vi "emi_ Set VIs Graphs Background .vi"(5 "VI Refnum(This vi)":refnum<vi>, 9 "error in (no error)":errorcluster) -> (6 "VI Refnum":refnum<vi>, 10 "error out":errorcluster)   [LabVIEW 2011]
doc: "Describe...\n\n\nIf no VI ref in, then the VI containing this VI is used.\nIf VI has multiple panes, only the first pane will be used.\n\nOn error in: Does not run."
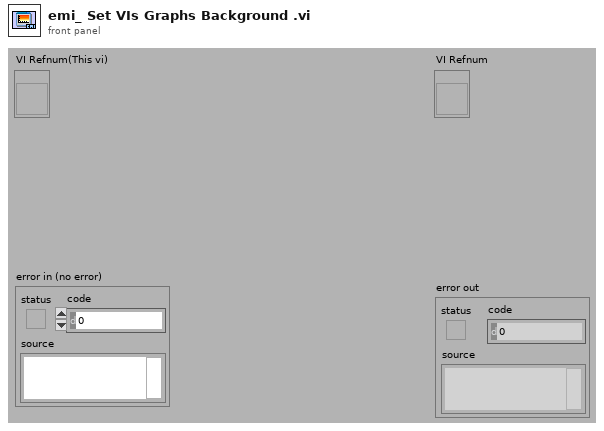
[diagram p1: front panel]
types:
  T1 = typedef "emi_System Colors.ctl" = cluster{"Main Top Panels":T2, "Main Botom Panels":T2, "Graphs":T2, "Dialogs":T2}
  T2 = typedef "_emi_ Color defenition.ctl" = cluster{"Type":T3, "Dark/Primary Color":u32, "Light/Secondary Color":u32, "Extra Color":u32}
  T3 = typedef "emi_List Of Graphix.ctl" = enum16{"FlatColor", "SharpGrad", "ShallowGrad", "GlasGradBord", "GlasGrad", "GlasGradBord 2"}
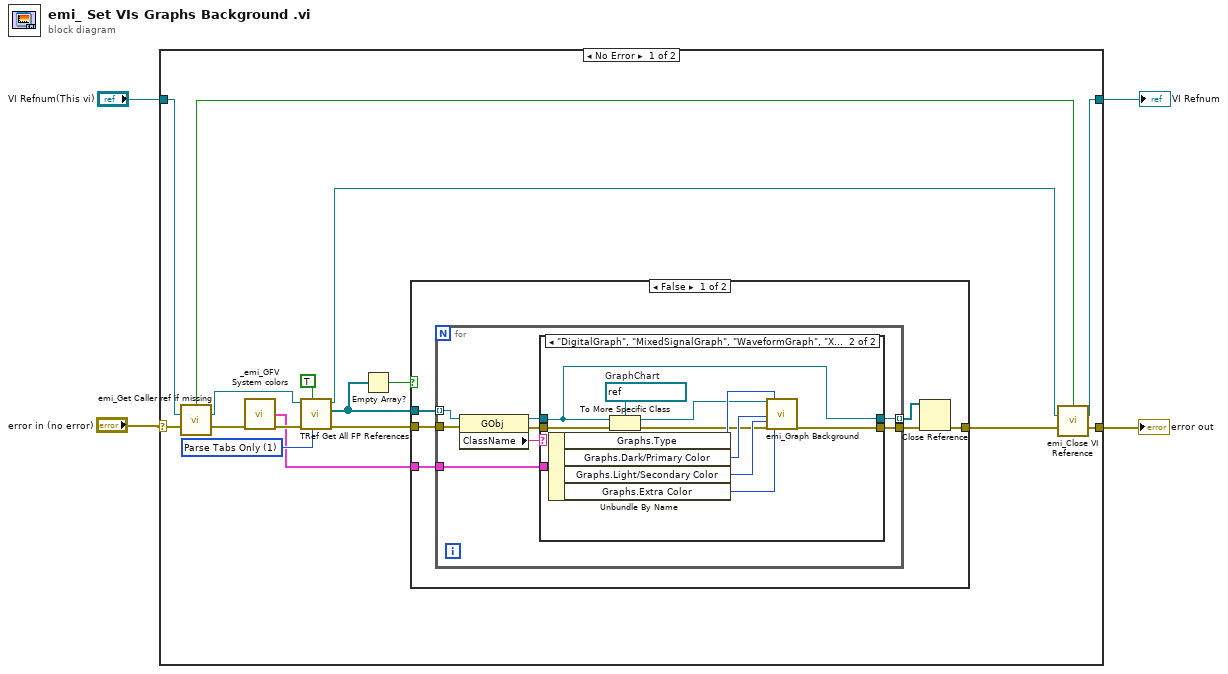
[diagram p0: block diagram]
diagram:
  n1 = case shown="No Error" "error in (no error)" {
    selector: "error in (no error)" -> [w19 w50]
    tunnel: [w17 w50] -> w4
    tunnel: "VI Refnum(This vi)" -> [w18 w49]
    tunnel: [w16 w49] -> w2
    frame No Error {
      w15 = u16 1 items=["Parse All", "Parse Tabs Only"] ("Parsing Rule")
      n2 = call "emi_Get Caller ref if missing.vi"("VI Refnum(Calling VI)"=w18, "error in (no error)"=w19) -> ("Ref Generated"=w20:bool, "VI Refnum Out"=w8:refnum<vi>, "error out"=w7:errorcluster)  [unwired: 11 in]
      n3 = call "_emi_GFV System colors.vi"("error in (no error)"=w7) -> ("System background out"=w9:T1, "error out"=w10:errorcluster)  [unwired: 13 in]
      n4 = call <vilib>:"TRef Get All FP References.vi"("Parsing Rule"=w15, "Ignore Decorations?"=TRUE, "error in (no error)"=w10, "VI Refnum"=w8) -> ("error out"=w11:errorcluster, "All FP Objects"=w12:refnum<vi>[], "dup VI Refnum"=w5:refnum<vi>)  [unwired: 3 in, 2 out]
      n5 = Empty Array?(array=w12) -> (empty?=w13:bool)
      n6 = case shown="False" w13 {
        tunnel: w12 -> [w26 _]
        tunnel: w11 -> [w25 w48]
        tunnel: w9 -> [w24 _]
        tunnel: [w21 w48] -> w6
        frame False {
          n7 = for {
            tunnel: w26 -> [w33] mode=indexing
            tunnel: w25 -> [w34]
            tunnel: w24 -> [w29]
            tunnel: [w28] -> w23
            tunnel: [w27] -> w22 mode=indexing
            n8 = property class="GObj"(reference=w33, error in=w34) -> (reference out=w30:refnum<vi>, error out=w31:errorcluster, "ClassName"=w32:string)
            n9 = case shown="\"DigitalGraph\", \"MixedSignalGraph\", \"WaveformGraph\", \"XYGraph\"" w32 {
              tunnel: w31 -> [w36 w47]
              tunnel: w30 -> [w35 w37]
              tunnel: w29 -> [_ w46]
              tunnel: [w36 w41] -> w28
              tunnel: [w35 w37] -> w27
              frame Default {
              }
              frame "DigitalGraph", "MixedSignalGraph", "WaveformGraph", "XYGraph" {
                w39 = refnum<vi> refnum  # GraphChart
                n10 = Unbundle By Name(w46) -> ("Graphs.Type"=w45:T3, "Graphs.Dark/Primary Color"=w44:u32, "Graphs.Light/Secondary Color"=w43:u32, "Graphs.Extra Color"=w42:u32)
                n11 = To More Specific Class(target class=w39, reference=w37, error in=w47) -> (specific class reference=w38:refnum<vi>, error out=w40:errorcluster)
                n12 = call "emi_Graph Background.vi"("Graph Refnum"=w38, "Dark(Black)"=w44, "Light(White)"=w43, "error in"=w40, "Graphic Type(FlatColor)"=w45, "Grid(Black)"=w42) -> ("error out"=w41:errorcluster)  [unwired: 12 in, 1 out]
              }
            }
          }
          n13 = Close Reference(reference=w22, error in (no error)=w23) -> (error out=w21:errorcluster)
        }
        frame True {
        }
      }
      n14 = call "emi_Close VI Reference.vi"("Close ref?(T)"=w20, "VI Refnum"=w5, "error in (no error)"=w6) -> ("VI Refnum Out"=w16:refnum<vi>, "error out"=w17:errorcluster)  [unwired: 11 in]
    }
    frame Error {
    }
  }
  "error out" <- w4
  "VI Refnum" <- w2
